vi "曲线拟合.vi"() -> ()   [LabVIEW 2018]
uses:
  <vilib>/Analysis/NI_AALPro.lvlib
  <vilib>/Analysis/NI_AALBase.lvlib
panel:
  in  "samples":i32=128 caption="采样"
  in  "停止":bool
  out "mean squared error":dynamicdata(graph) caption="均方误差"
  out "residual":dynamicdata(graph) caption="残差"
  out "best fit":dynamicdata(graph) caption="最佳拟合"
  in  "amplitude":dbl=1.0 caption="幅值" format="%0.2f"
  in  "frequency":dbl=10.0 caption="频率" format="%0.2f"
  in  "signal type":T1(ring) caption="信号类型"
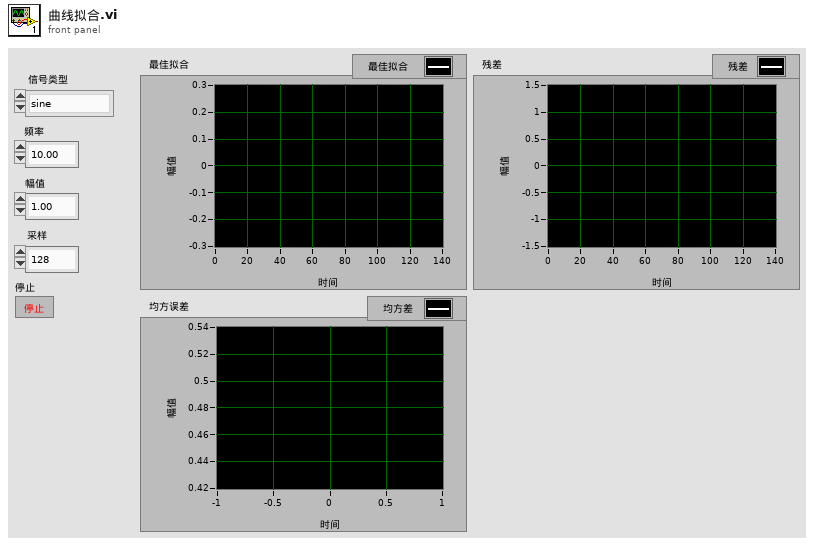
[diagram p1: front panel]
types:
  T1 = enum16{"sine", "cosine", "triangle", "square", "sawtooth", "increasing ramp", "decreasing ramp"}
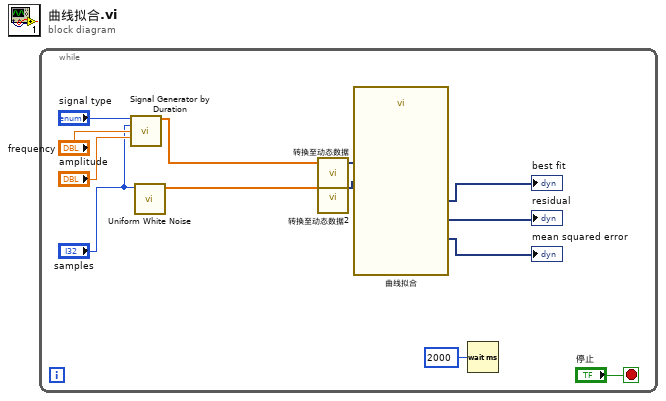
[diagram p0: block diagram]
diagram:
  n1 = while {
    stop <- "停止" stop-if-true
    n2 = call <vilib>:"Signal Generator by Duration.vi"("signal type"="signal type", "# of samples"="samples", "frequency"="frequency", "amplitude"="amplitude") -> ("signal"=w10:dbl[])  [unwired: 8 in, 3 out]
    n3 = call <vilib>:"Uniform White Noise.vi"("samples"="samples") -> ("uniform white noise"=w8:dbl[])  [unwired: 9 in, 1 out]
    n4 = call "转换至动态数据"("Array"=w10) -> ("Dynamic Data Type"=w9:dynamicdata)  [unwired: 3 in]
    n5 = call "转换至动态数据2"("Array"=w8) -> ("Dynamic Data Type"=w7:dynamicdata)  [unwired: 3 in]
    n6 = call "曲线拟合"("Locations"=w7, "Signals"=w9) -> ("mean squared error"=→"mean squared error":dynamicdata, "residual"=→"residual":dynamicdata, "best fit"=→"best fit":dynamicdata)  [unwired: 5 in, 2 out]
    n7 = Wait (ms)(milliseconds to wait=u32 2000 ("等待时间（毫秒）")) -> ()  [unwired: 1 out]
  }
